vi "Append Common Headers.vi"(8 "Error In":errorcluster, 11 "Nest Config":T1) -> (0 "Error Out":errorcluster, 3 "Nest Config":T1)   [LabVIEW 2013, in "LVH-Nest.lvlib"]
doc: "Load common HTTP headers for Nest communication."
uses:
  LVH-Nest.lvlib
  Type Defs/Nest Config.ctl
  <vilib>/httpClient/ClientHandle.ctl
  Type Defs/Session Data.ctl
  <vilib>/httpClient/LabVIEWHTTPClient.lvlib
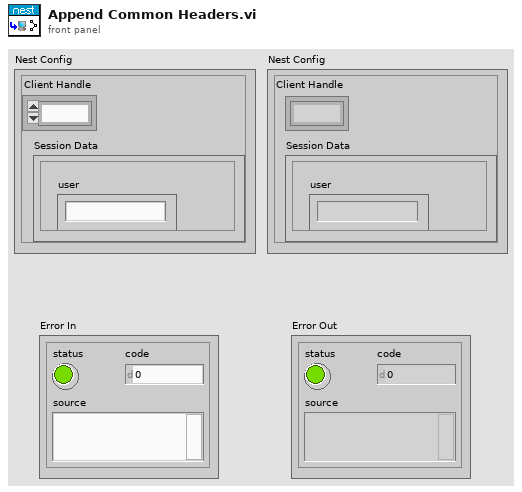
[diagram p1: front panel]
types:
  T1 = typedef "LVH-Nest.lvlib/Nest Config.ctl" = cluster{"Client Handle":T2, "Session Data":T3}
  T2 = typedef "LabVIEWHTTPClient.lvlib/ClientHandle.ctl" = refnum<k1>
  T3 = typedef "LVH-Nest.lvlib/Session Data.ctl" = cluster{"is_superuser":bool, "is_staff":bool, "urls":cluster{"transport_url":string, "rubyapi_url":string, "weather_url":string, "log_upload_url":string, "support_url":string}, "limits":cluster{"thermostats_per_structure":u32, "structures":u32, "thermostats":u32, "smoke_detectors":u32, "smoke_detectors_per_structure":u32}, "access_token":string, "userid":string, "expires_in":string, "email":string, "user":string, "language":string}
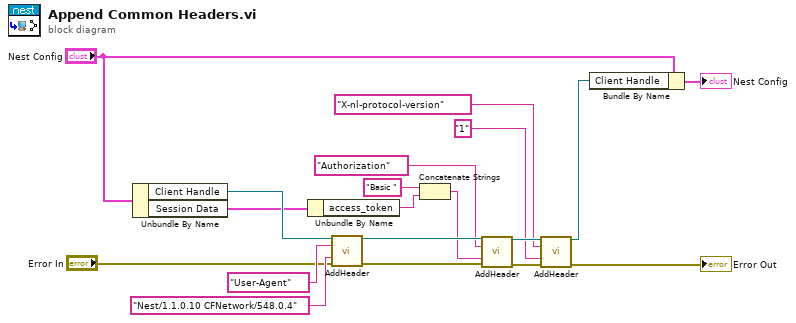
[diagram p0: block diagram]
diagram:
  n1 = Unbundle By Name("Nest Config") -> ("Client Handle"=w19:T2, "Session Data"=w10:T3)
  n2 = Unbundle By Name(w10) -> ("access_token"=w12:string)
  n3 = call <vilib>:"AddHeader.vi"("client handle"=w19, "header"="User-Agent", "value"="Nest/1.1.0.10 CFNetwork/548.0.4", "error in (no error)"="Error In") -> ("client handle out"=w15:T2, "error out"=w14:errorcluster)  [unwired: 10 in]
  n4 = Concatenate Strings("Basic " ("string"), w12) -> (w9:string)
  n5 = call <vilib>:"AddHeader.vi"("client handle"=w15, "header"="Authorization", "value"=w9, "error in (no error)"=w14) -> ("client handle out"=w8:T2, "error out"=w7:errorcluster)  [unwired: 10 in]
  n6 = call <vilib>:"AddHeader.vi"("client handle"=w8, "header"="X-nl-protocol-version", "value"="1", "error in (no error)"=w7) -> ("client handle out"=w1:T2, "error out"=→"Error Out":errorcluster)  [unwired: 10 in]
  n7 = Bundle By Name(cluster="Nest Config", "Client Handle"=w1) -> (→"Nest Config":T1)
